vi "GVMWHorst.vi"() -> ()   [LabVIEW 2010]
panel:
  in  "MWHorst":dbl[](array[numeric])
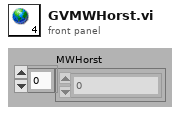
[diagram p1: front panel]
diagram:
